vi "GUILaptop.vi"() -> ()   [LabVIEW 2016]
uses:
  <vilib>/dex/Stream Element Allocation Mode.ctl
panel:
  in  "Dial":dbl(knob) scale=0.0..1.0
  out "element 7":dbl
  out "element 6":dbl
  out "element 5":dbl
  out "element 4":dbl
  out "element 3":dbl
  out "element 2":dbl
  out "element":dbl
  in  "stop":bool
  # "Minimum"
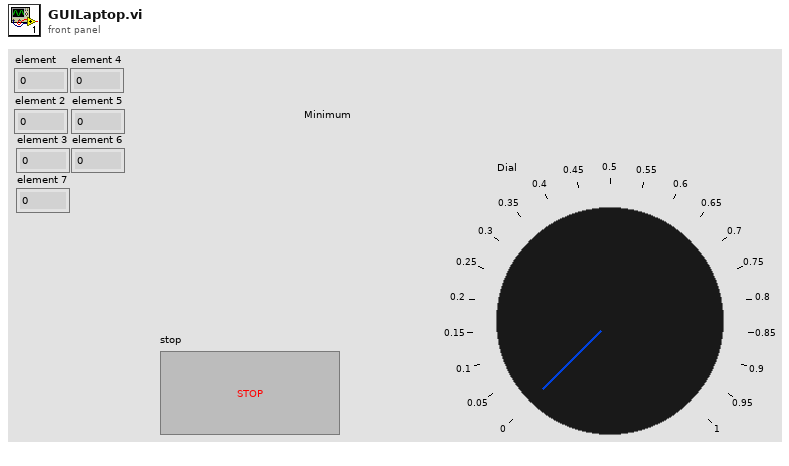
[diagram p1: front panel]
types:
  T1 = typedef "Stream Element Allocation Mode.ctl" = u32
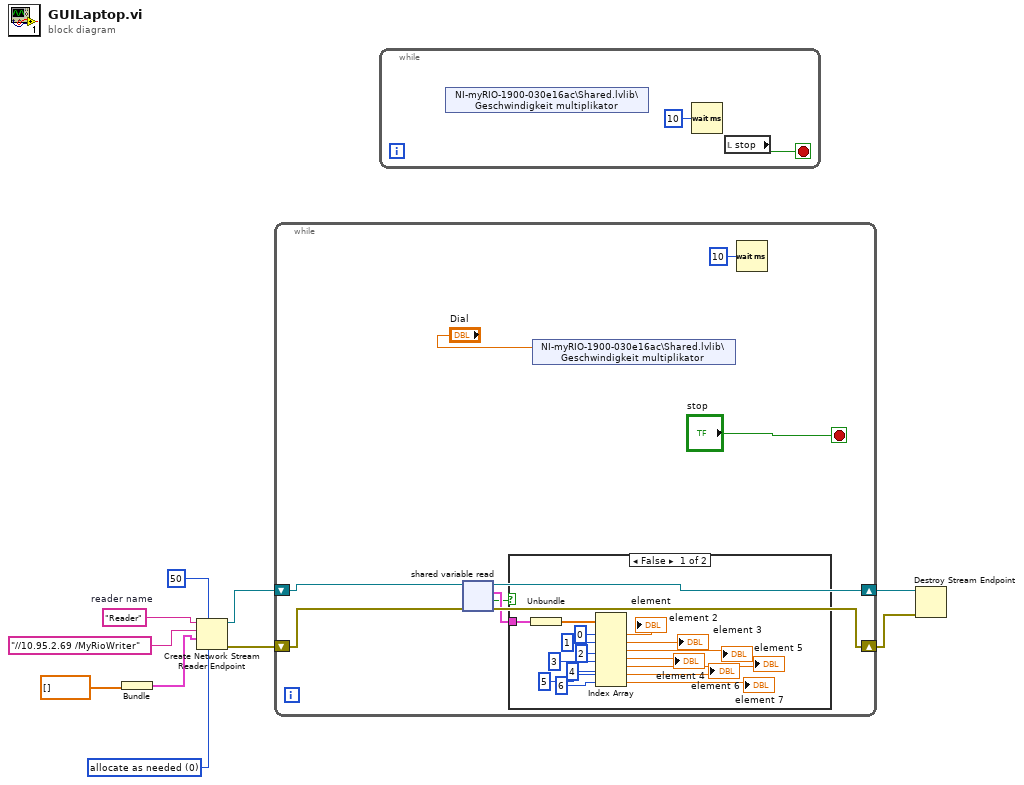
[diagram p0: block diagram]
diagram:
  w5 = T1 0 items=["allocate as needed", "pre-allocate"] ("element allocation mode")
  w4 = "Reader"  # reader name
  n1 = Bundle(dbl[] []) -> (w1:cluster{dbl[]})  [unwired: 1 in]
  n2 = Create Network Stream Reader Endpoint(6:w5, 7:50 ("reader buffer size"), 9:w1, 10:"//10.95.2.69 /MyRioWriter" ("writer url"), 11:w4) -> (0:w8:errorcluster, 3:w9:refnum<k21>)  [unwired: 2 in]
  n3 = while {
    shift-right: [w16] -> w7
    shift-left: w9 -> [w18]
    shift-right: [w15] -> w6
    shift-left: w8 -> [w17]
    stop <- "stop" stop-if-true
    n4 = shared-variable-read(w18, w17) -> (w16:refnum<k21>, w15:errorcluster, w12:bool, w13:cluster{dbl[]})  [unwired: 1 in]
    n5 = case shown="False" w12 {
      tunnel: w13 -> [w35 _]
      frame False {
        n6 = Unbundle(w35) -> (w20:dbl[])
        n7 = Index Array(array=w20, index #1=0 ("index"), index #2=1 ("index"), index #3=2 ("index"), index #4=3 ("index"), index #5=4 ("index"), index #6=5 ("index"), index #7=6 ("index")) -> (element #1=→"element":dbl, element #2=→"element 2":dbl, element #3=→"element 3":dbl, element #4=→"element 4":dbl, element #5=→"element 5":dbl, element #6=→"element 6":dbl, element #7=→"element 7":dbl)
      }
      frame True {
      }
    }
    n8 = shared-variable "NI-myRIO-1900-030e16ac\\Shared.lvlib\\Geschwindigkeit multiplikator"("Dial") -> ()  [unwired: 1 in, 1 out]
    n9 = Wait (ms)(milliseconds to wait=u32 10) -> ()  [unwired: 1 out]
  }
  n10 = while {
    stop <- w36 stop-if-true
    n11 = shared-variable "NI-myRIO-1900-030e16ac\\Shared.lvlib\\Geschwindigkeit multiplikator"() -> ()  [unwired: 1 in, 2 out]
    n12 = Wait (ms)(milliseconds to wait=u32 10) -> ()  [unwired: 1 out]
    n13 = local read "stop"() -> (w36:bool)
  }
  n14 = Destroy Stream Endpoint(8:w6, 11:w7) -> ()  [unwired: 1 out]
